vi "Receive.vi"(6 "Timeout ms":i32=1, 7 "UDP Input":T1) -> (0 "Error Out":errorcluster, 1 "Received Data":string, 2 "Did Receive":bool, 3 "UDP Output":T1)   [LabVIEW 2019]
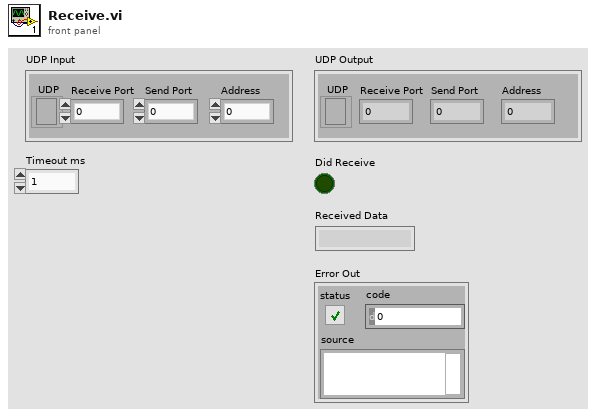
[diagram p1: front panel]
types:
  T1 = cluster{"UDP":refnum<k16>, "Receive Port":i32, "Send Port":i32, "Address":i64}
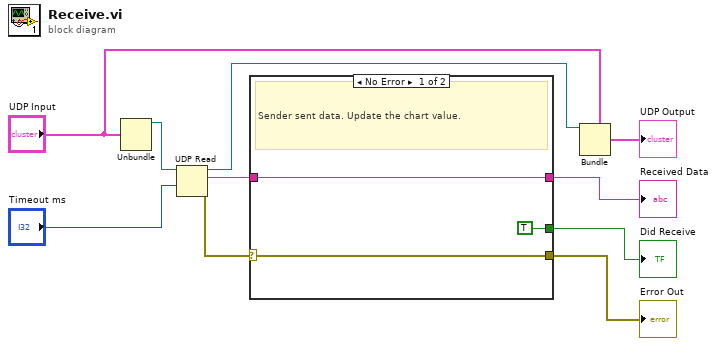
[diagram p0: block diagram]
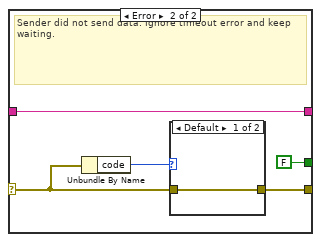
[diagram p2: hidden frame]
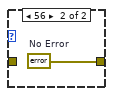
[diagram p3: hidden frame]
diagram:
  n1 = Unbundle("UDP Input") -> ("UDP"=w6:refnum<k16>)  [unwired: 3 out]
  n2 = UDP Read(connection ID=w6, timeout ms (25000)="Timeout ms") -> (data out=w10:string, error out=w8:errorcluster, 3:w5:refnum<k16>)  [unwired: 2 in, 2 out]
  n3 = case shown="No Error" w8 {
    selector: w8 -> [w13 w17]
    tunnel: w10 -> [w12 w15]
    tunnel: [w13 w16] -> w9
    tunnel: [w12 w15] -> w2
    tunnel: [TRUE FALSE] -> w1
    frame No Error {
      # "Sender sent data. Update the chart value."
    }
    frame Error {
      # "Sender did not send data. Ignore timeout error and keep waiting."
      n4 = Unbundle By Name(w17) -> ("code"=w18:i32)
      n5 = case shown="Default" w18 {
        tunnel: w17 -> [w19 _]
        tunnel: [w19 w20] -> w16
        frame Default {
        }
        frame 56 {
          w20 = errorcluster {"status"=FALSE, "code"=0, "source"=""}  # No Error
        }
      }
    }
  }
  "Error Out" <- w9
  "Received Data" <- w2
  "Did Receive" <- w1
  n6 = Bundle(cluster="UDP Input", "UDP"=w5) -> (→"UDP Output":T1)  [unwired: 3 in]
